vi "USB205_SetVoltage.vi"() -> ()   [LabVIEW 2024]
uses:
  <instrlib>/ULx/Create Channel.llb/ULx Create Channel (AO-Voltage-Basic).vi
  <instrlib>/ULx/Write.llb/ULx Write (Analog 1D DBL 1Chan 1Samp).vi
panel:
  in  "Voltage2":dbl
  out "number of samples written per channel 2":u32
  out "error out":errorcluster
  out "number of samples written per channel":u32
  in  "Voltage1":dbl
  in  "stop":bool
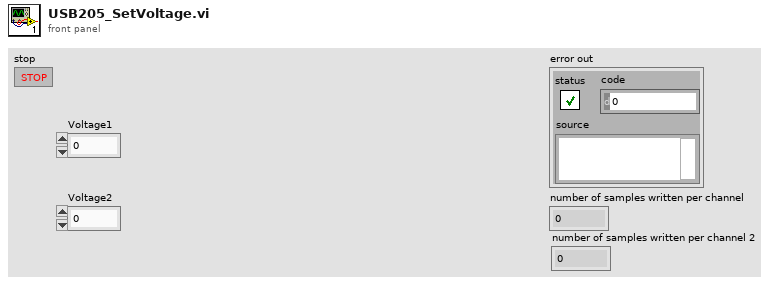
[diagram p1: front panel]
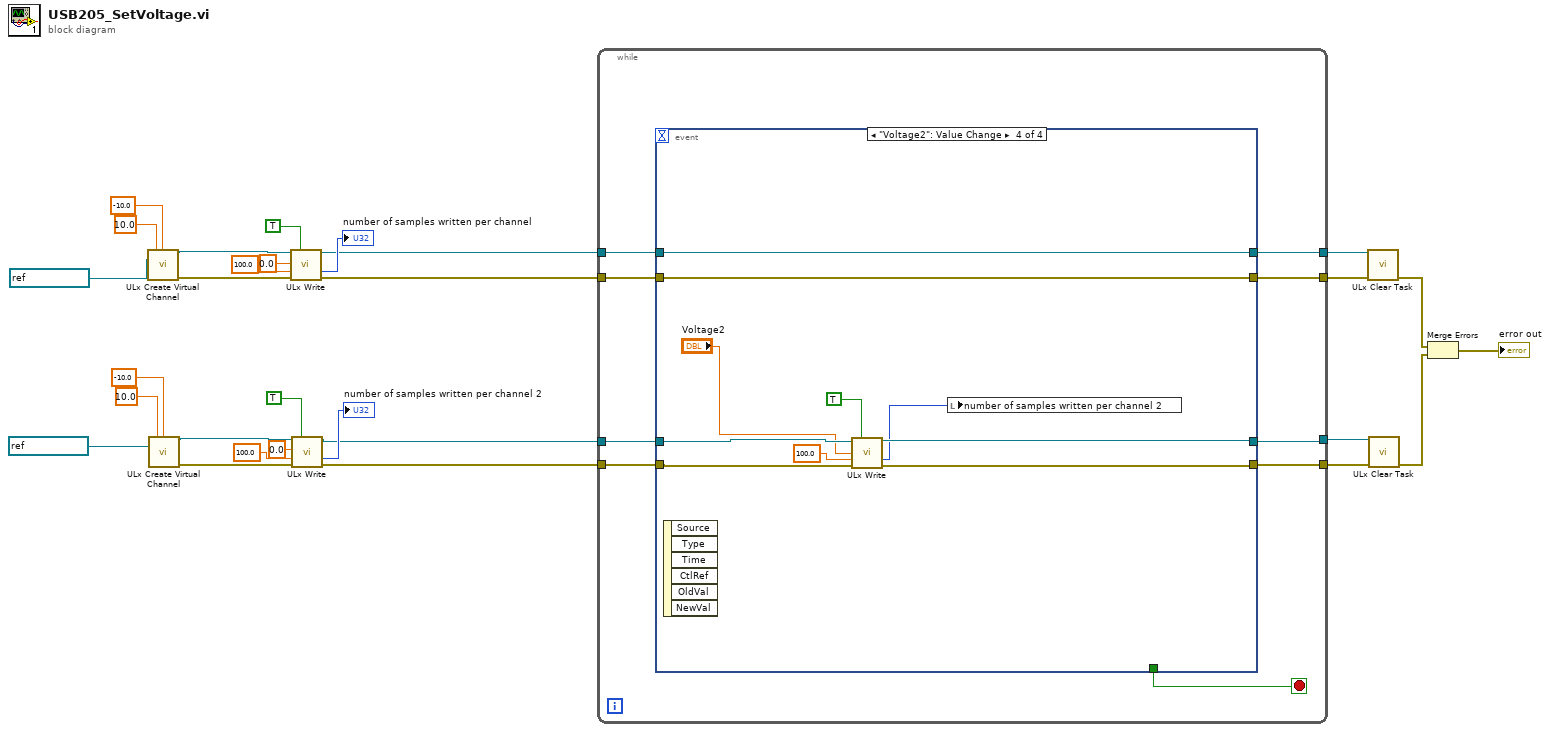
[diagram p0: block diagram]
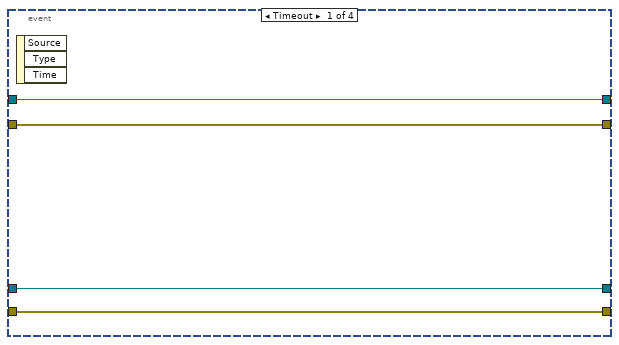
[diagram p2: hidden frame]
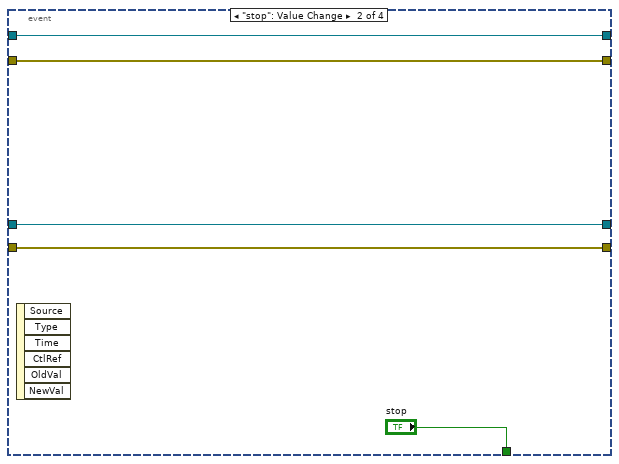
[diagram p3: hidden frame]
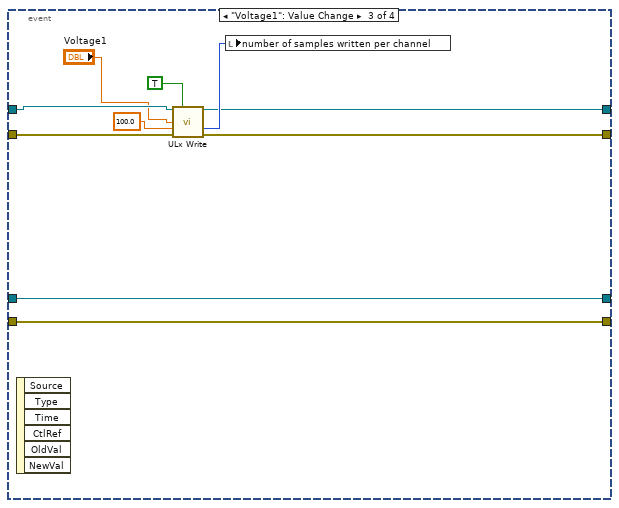
[diagram p4: hidden frame]
diagram:
  n1 = call-poly <instrlib>:"ULx Create Virtual Channel.vi"("maximum value"=10.0, "minimum value"=-10.0, "physical channels"=refnum<k21> "Dev0/Ao3") -> ("task out"=w29:refnum<k24>, "error out"=w28:errorcluster)  [unwired: 11 in]
  n2 = call-poly <instrlib>:"ULx Create Virtual Channel.vi"("maximum value"=10.0, "minimum value"=-10.0, "physical channels"=refnum<k21> "Dev0/Ao5" ("physical channels 2")) -> ("task out"=w20:refnum<k24>, "error out"=w21:errorcluster)  [unwired: 11 in]
  n3 = call-poly <instrlib>:"ULx Write.vi"("task in"=w29, "auto start"=TRUE, "data"=0.0, "timeout"=100.0, "error in"=w28) -> ("task out"=w8:refnum<k24>, "number of samples written per channel"=→"number of samples written per channel":u32, "error out"=w7:errorcluster)  [unwired: 8 in]
  n4 = call-poly <instrlib>:"ULx Write.vi"("task in"=w20, "auto start"=TRUE, "data"=0.0, "timeout"=100.0, "error in"=w21) -> ("task out"=w6:refnum<k24>, "number of samples written per channel"=→"number of samples written per channel 2":u32, "error out"=w5:errorcluster)  [unwired: 8 in]
  n5 = while {
    tunnel: w8 -> [w34]
    tunnel: w7 -> [w35]
    tunnel: w6 -> [w36]
    tunnel: w5 -> [w37]
    tunnel: [w33] -> w4
    tunnel: [w32] -> w3
    tunnel: [w31] -> w2
    tunnel: [w30] -> w1
    stop <- w38 stop-if-true
    n6 = event shown="[3] \"Voltage2\": Value Change" {
      selector: _ -> [_ _ _ _]
      dyn-events: _ -> [_ _ _ _]
      timeout: _ -> [_ _ _ _]
      tunnel: [_ "stop" _ _] -> w38
      tunnel: w37 -> [w39 w43 w50 w63]
      tunnel: w36 -> [w40 w44 w51 w62]
      tunnel: w35 -> [w41 w45 w54 w66]
      tunnel: w34 -> [w42 w46 w53 w67]
      tunnel: [w42 w46 w48 w67] -> w33
      tunnel: [w41 w45 w49 w66] -> w32
      tunnel: [w40 w44 w51 w60] -> w31
      tunnel: [w39 w43 w50 w59] -> w30
      event Timeout {
        n7 = event-data() -> ()  [unwired: 1 in, 3 out]
      }
      event "stop": Value Change {
        n8 = event-data() -> ()  [unwired: 1 in, 6 out]
      }
      event "Voltage1": Value Change {
        n9 = event-data() -> ()  [unwired: 1 in, 6 out]
        n10 = call-poly <instrlib>:"ULx Write.vi"("task in"=w53, "auto start"=TRUE, "data"="Voltage1", "timeout"=100.0, "error in"=w54) -> ("task out"=w48:refnum<k24>, "number of samples written per channel"=w55:u32, "error out"=w49:errorcluster)  [unwired: 8 in]
        n11 = local write "number of samples written per channel"(w55) -> ()
      }
      event "Voltage2": Value Change {
        n12 = event-data() -> ()  [unwired: 1 in, 6 out]
        n13 = call-poly <instrlib>:"ULx Write.vi"("task in"=w62, "auto start"=TRUE, "data"="Voltage2", "timeout"=100.0, "error in"=w63) -> ("task out"=w60:refnum<k24>, "number of samples written per channel"=w58:u32, "error out"=w59:errorcluster)  [unwired: 8 in]
        n14 = local write "number of samples written per channel 2"(w58) -> ()
      }
    }
  }
  n15 = call <instrlib>:"ULx Clear Task.vi"("task in"=w4, "error in"=w3) -> ("error out"=w18:errorcluster)  [unwired: 13 in]
  n16 = call <instrlib>:"ULx Clear Task.vi"("task in"=w2, "error in"=w1) -> ("error out"=w17:errorcluster)  [unwired: 13 in]
  n17 = Merge Errors(w18, w17) -> (→"error out":errorcluster)
